vi "VrmVISACommandAndResponse.vi"(8 "error in (no error)":errorcluster, 10 "Command":string, 11 "VISA resource name in":refnum<visa-resource-name>) -> (0 "error out":errorcluster, 2 "Response":string, 3 "VISA resource name out":refnum<visa-resource-name>)   [LabVIEW 2021]
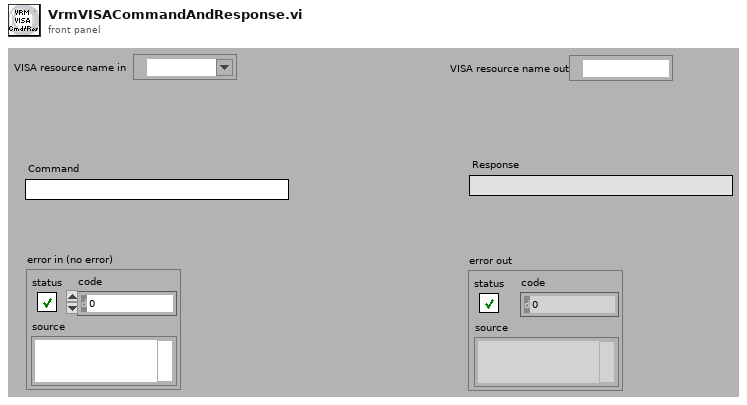
[diagram p1: front panel]
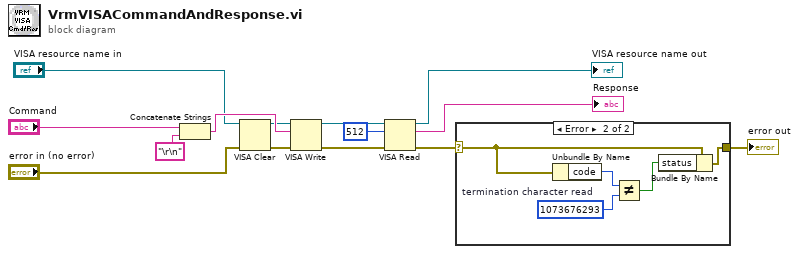
[diagram p0: block diagram]
diagram:
  n1 = Concatenate Strings("Command", "\r\n" ("string")) -> (w11:string)
  n2 = VISA Clear(VISA resource name="VISA resource name in", error in (no error)="error in (no error)") -> (VISA resource name out=w7:refnum<visa-resource-name>, error out=w8:errorcluster)
  n3 = VISA Write(VISA resource name=w7, write buffer=w11, error in (no error)=w8) -> (VISA resource name out=w13:refnum<visa-resource-name>, error out=w14:errorcluster)  [unwired: 1 out]
  n4 = VISA Read(VISA resource name=w13, byte count=u32 512, error in (no error)=w14) -> (VISA resource name out=→"VISA resource name out":refnum<visa-resource-name>, read buffer=→"Response":string, error out=w2:errorcluster)  [unwired: 1 out]
  n5 = case shown="Error" w2 {
    selector: w2 -> [w15 w18]
    tunnel: [w15 w16] -> w1
    frame No Error {
    }
    frame Error {
      w20 = 1073676293  # termination character read
      n6 = Unbundle By Name(w18) -> ("code"=w19:i32)
      n7 = Not Equal?(x=w19, y=w20) -> (x != y?=w17:bool)
      n8 = Bundle By Name(cluster=w18, "status"=w17) -> (w16:errorcluster)
    }
  }
  "error out" <- w1
